vi "variant2Attributes.vi"(0 "HGV_PVBase":refnum<class "HGF_SVCommand.lvclass">, 2 "rawData":variant, 3 "typeDescriptor":string, 5 "error in (no error)":errorcluster) -> (14 "HGV_PVBase":refnum<class "HGF_SVCommand.lvclass">, 15 "no link":bool, 16 "Parameter":variant, 17 "typeDescriptor":string, 19 "error out":errorcluster)   [LabVIEW 2012, in "HGF_SV.lvlib" / "HGF_SVCommand.lvclass"]
doc: "Convert raw data value of variant to variant attributes Pn, n=0,1,2,..."
uses:
  HGF_SVCommand.lvclass
  HGF_BaseClasses/HGF_PVSubscriber/HGF_PVSubscriber.lvclass
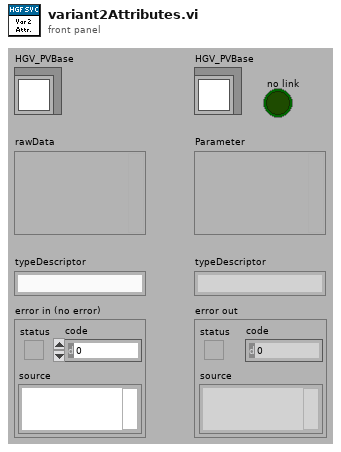
[diagram p1: front panel]
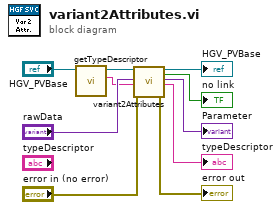
[diagram p0: block diagram]
diagram:
  n1 = call-dynamic "getTypeDescriptor.vi"("HGF_SVCommand.lvclass in"="HGV_PVBase") -> ("typeDescriptor"=w1:string, "HGF_SVCommand.lvclass out"=w3:refnum<class "HGF_SVCommand.lvclass">)  [unwired: 1 in, 8 out]
  n2 = call-parent "variant2Attributes.vi"("HGV_PVBase"=w3, "rawData"="rawData", "typeDescriptor"=w1, "error in (no error)"="error in (no error)") -> ("HGV_PVBase"=→"HGV_PVBase":refnum<class "HGF_SVCommand.lvclass">, "no link"=→"no link":bool, "Parameter"=→"Parameter":variant, "typeDescriptor"=→"typeDescriptor":string, "error out"=→"error out":errorcluster)  [unwired: 11 out]
